vi "显示场景面板.vi"(8 "node":T1(array[cluster]), 10 "数目":i32, 11 "节点引用数组":refnum<vi>[](array[refnum])) -> ()   [LabVIEW 2019]
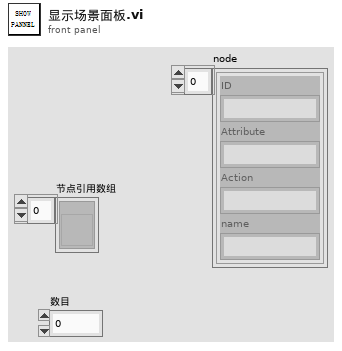
[diagram p1: front panel]
types:
  T1 = cluster{"ID":string, "Attribute":string, "Action":string, "name":string}[]
  T2 = cluster{"ID":u8, "type":string, "flag":string, "name":string, "Act":cluster{"Attribute":string, "Action":string, "Value":dbl}}
  T3 = cluster{"ID":string, "Attribute":string, "Action":string, "name":string}
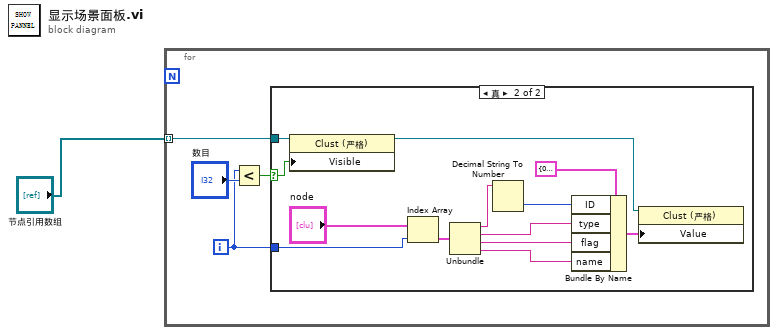
[diagram p0: block diagram]
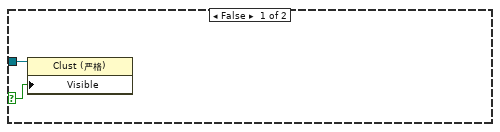
[diagram p2: hidden frame]
diagram:
  n1 = for {
    tunnel: "节点引用数组" -> [w3] mode=indexing
    i -> [w2]
    n2 = Less?(x=w2, y="数目") -> (x < y?=w4:bool)
    n3 = case shown="真" w4 {
      selector: w4 -> [w7 w20]
      tunnel: w3 -> [w6 w19]
      tunnel: w2 -> [_ w9]
      frame False {
        n4 = property class="Clust (严格)"(reference=w6, "Visible"=w7) -> ()  [unwired: 1 in, 2 out]
      }
      frame True {
        n5 = property class="Clust (严格)"(reference=w19, "Visible"=w20) -> (reference out=w18:refnum<vi>)  [unwired: 1 in, 1 out]
        n6 = Index Array(array="node", index=w9) -> (element=w8:T3)
        n7 = Unbundle(w8) -> ("ID"=w16:string, "Attribute"=w14:string, "Action"=w13:string, "name"=w12:string)
        n8 = Decimal String To Number(string=w16) -> (number=w15:i32)  [unwired: 2 in, 1 out]
        n9 = Bundle By Name(cluster=T2 {"ID"=0, "type"="", "flag"="", "name"="", "Act"={"Attribute"="", "Action"="", "Value"=0.0}} ("值"), "ID"=w15, "type"=w14, "flag"=w13, "name"=w12) -> (w11:T2)
        n10 = property class="Clust (严格)"(reference=w18, "Value"=w11) -> ()  [unwired: 1 in, 2 out]
      }
    }
  }
